vi "buildLogEntry.vi"(8 "error in (no error)":errorcluster, 9 "command line":string, 10 "standard output":string) -> (0 "error out":errorcluster, 2 "Log Entry":string)   [LabVIEW 2013]
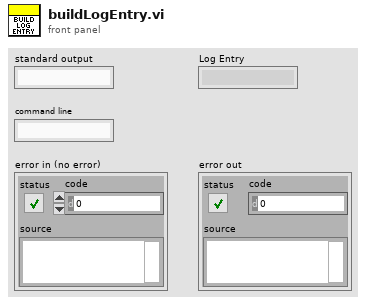
[diagram p1: front panel]
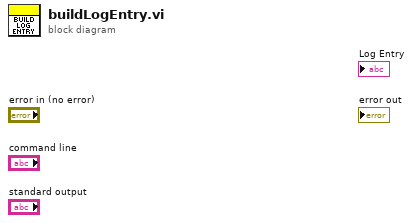
[diagram p0: block diagram]
diagram:
